vi "Read Atts.vi"(8 "error in (no error)":errorcluster, 11 "keysight in":refnum<class "keysight.lvclass">) -> (0 "error out":errorcluster, 1 "IF_Band":dbl, 2 "Stop":dbl, 3 "keysight out":refnum<class "keysight.lvclass">, 4 "Points":i32, 5 "Start":dbl)   [LabVIEW 2015, in "keysight.lvclass"]
uses:
  keysight.lvclass
  keysight.lvclass/keysight.ctl
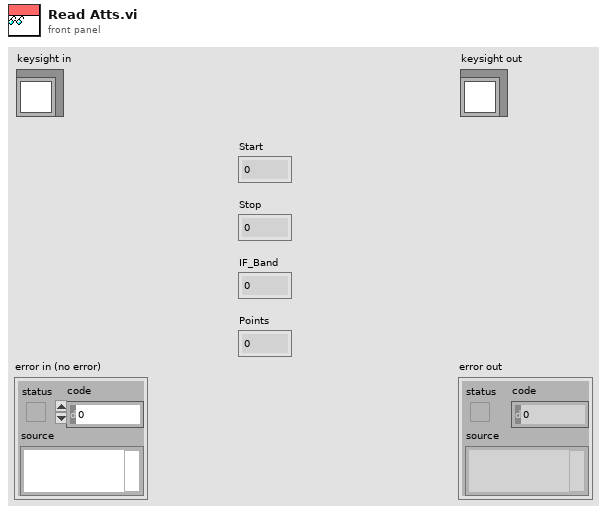
[diagram p1: front panel]
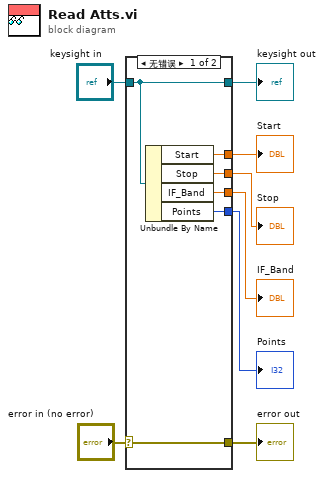
[diagram p0: block diagram]
diagram:
  n1 = case shown="无错误" "error in (no error)" {
    selector: "error in (no error)" -> [w14 w16]
    tunnel: [w14 w16] -> w7
    tunnel: "keysight in" -> [w9 w15]
    tunnel: [w13 _] -> w5
    tunnel: [w12 _] -> w4
    tunnel: [w11 _] -> w3
    tunnel: [w10 _] -> w2
    tunnel: [w9 w15] -> w1
    frame No Error {
      n2 = Unbundle By Name(w9) -> ("Start"=w13:dbl, "Stop"=w12:dbl, "IF_Band"=w11:dbl, "Points"=w10:i32)
    }
    frame Error {
    }
  }
  "error out" <- w7
  "keysight out" <- w1
  "Stop" <- w4
  "IF_Band" <- w3
  "Points" <- w2
  "Start" <- w5
